vi "Get Compiler Level.vi"(8 "error in (no error)":errorcluster, 11 "NI_AB_API_PPL in":refnum<class "NI_AB_API_PPL.lvclass">) -> (0 "error out":errorcluster, 2 "compiler Level":u32=1, 3 "NI_AB_API_PPL out":refnum<class "NI_AB_API_PPL.lvclass">)   [LabVIEW 2020, in "NI_AB_API_PPL.lvclass"]
uses:
  <vilib>/AppBuilder/AB_API/PPL/NI_AB_API_PPL.lvclass
  <vilib>/AppBuilder/AB_API/Targetfile/NI_AB_API_Targetfile.lvclass
  <vilib>/AppBuilder/AB_API/PPL/NI_AB_API_PPL.lvclass/NI_AB_API_PPL.ctl
panel:
  # "0: SSE2 optimization disabled\n1: SSE2 optimization enabled"
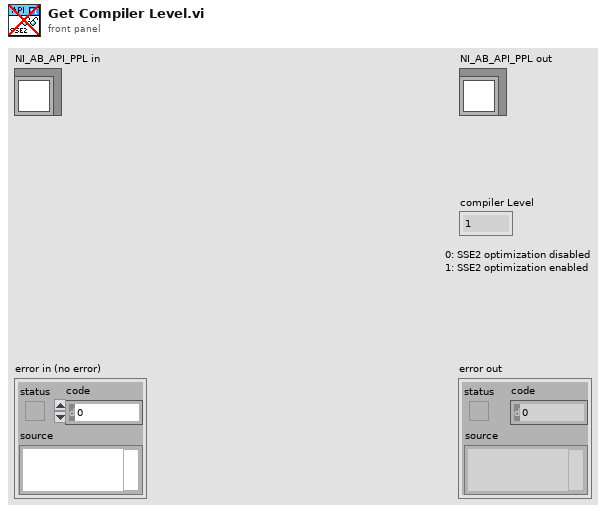
[diagram p1: front panel]
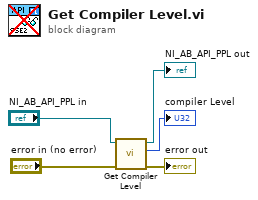
[diagram p0: block diagram]
diagram:
  n1 = call-parent "Get Compiler Level.vi"("error in (no error)"="error in (no error)", "NI_AB_API_Build in"="NI_AB_API_PPL in") -> ("error out"=→"error out":errorcluster, "compiler Level"=→"compiler Level":u32, "NI_AB_API_Build out"=→"NI_AB_API_PPL out":refnum<class "NI_AB_API_PPL.lvclass">)  [unwired: 7 in]
